vi "GetClusterElementByName(Variant).vi"(10 "ElementHierarchy":string[](array[string]), 11 "Cluster":variant) -> (2 "Found":bool, 3 "Element":variant)   [LabVIEW 2020, in "GetClusterElementByName.lvlib"]
uses:
  GetClusterElementByName.lvlib
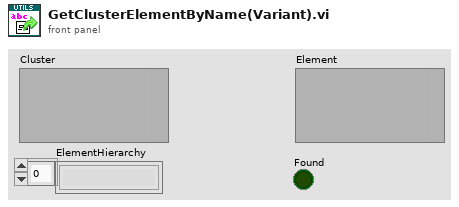
[diagram p1: front panel]
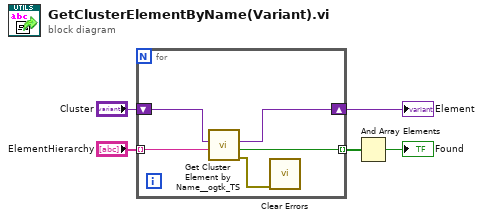
[diagram p0: block diagram]
diagram:
  n1 = for {
    tunnel: "ElementHierarchy" -> [w10] mode=indexing
    shift-right: [w9] -> w5
    shift-left: "Cluster" -> [w8]
    tunnel: [w7] -> w2 mode=indexing
    n2 = call "Get Cluster Element by Name__ogtk_TS.vi"("Element Name"=w10, "Cluster"=w8) -> ("error out"=w6:errorcluster, "found?"=w7:bool, "VElement"=w9:variant)  [unwired: 7 in]
    n3 = call <vilib>:"Clear Errors.vi"("error in (no error)"=w6) -> ()  [unwired: 5 in, 2 out]
  }
  "Element" <- w5
  n4 = And Array Elements(Boolean array=w2) -> (logical AND=→"Found":bool)
